vi "loadFileSystem.vi"(8 "error in (no error)":errorcluster, 10 "computer name":string) -> (0 "error out":errorcluster, 3 "FileSystem out":refnum<class "FileSystem.lvclass">)   [LabVIEW 2011, in "Tools.lvlib" / "Filing.lvlib" / "FileSystem.lvclass"]
uses:
  FileSystem.lvclass
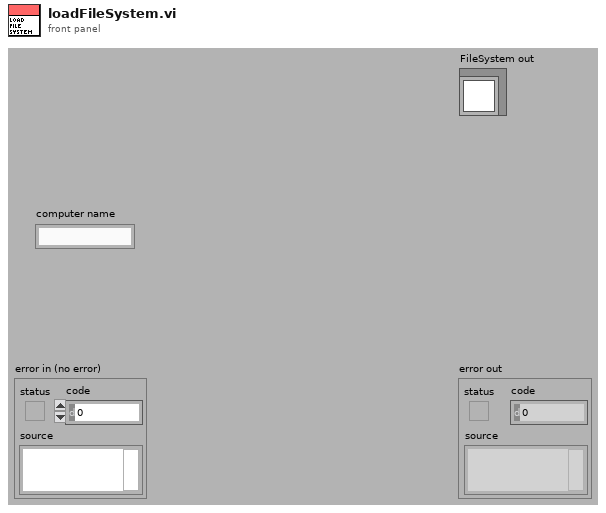
[diagram p1: front panel]
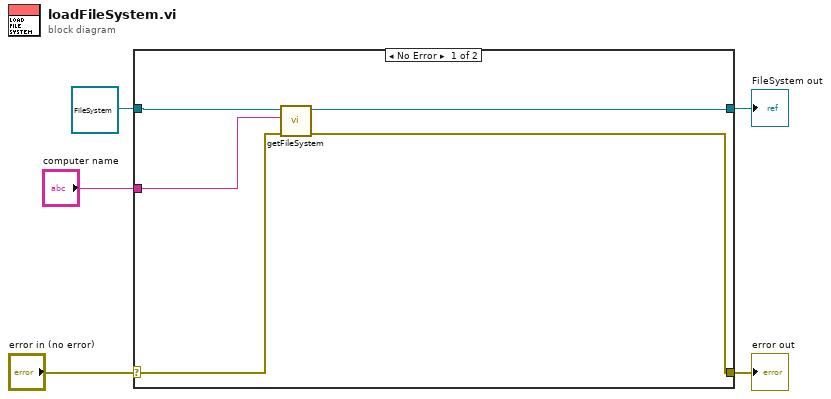
[diagram p0: block diagram]
diagram:
  n1 = case shown="No Error" "error in (no error)" {
    selector: "error in (no error)" -> [w8 w12]
    tunnel: [w7 w12] -> w4
    tunnel: [w6 w11] -> w2
    tunnel: refnum<class "FileSystem.lvclass"> refnum ("FileSystem in") -> [w10 w11]
    tunnel: "computer name" -> [w9 _]
    frame No Error {
      n2 = call "getFileSystem.vi"("error in (no error)"=w8, "computer"=w9, "FileSystem in"=w10) -> ("error out"=w7:errorcluster, "FileSystem out"=w6:refnum<class "FileSystem.lvclass">)  [unwired: 7 in]
    }
    frame Error {
    }
  }
  "error out" <- w4
  "FileSystem out" <- w2
